vi "DrawSubMenuItems.vi"(7 "Collection in":refnum<class "Collection.lvclass">, 8 "error in (no error)":errorcluster, 9 "Coords":T2, 10 "Tag":string, 11 "Menu in":refnum<class "Menu.lvclass">) -> (0 "error out":errorcluster, 1 "SubMenu":bool, 2 "SelectedArea":T1, 3 "Menu out":refnum<class "Menu.lvclass">, 4 "SelectedItemTag":string, 5 "Collection out":refnum<class "Collection.lvclass">, 6 "GlobalArea":T1)   [LabVIEW 2021, in "Menu.lvlib" / "Menu.lvclass"]
uses:
  Menu.lvclass
  Menu.lvclass/Menu.ctl
  Picture2D/src/Collection/Collection.lvclass
  Picture2D/src/Rectangle/Rectangle.lvclass
  Picture2D/src/Text/Text.lvclass
  Picture2D/src/Picture/Image.lvclass
  Picture2D/src/Point/Point.lvclass
  C:/GitHub/Picture2D/src/Polygone/Polygone.lvclass
  C:/GitHub/Picture2D/src/Shape/Shape.lvclass
  C:/GitHub/Picture2D/src/Picture2D/Picture2D.lvclass
  C:/GitHub/Picture2D/src/IDrawable/IDrawable.lvclass
  C:/GitHub/Picture2D/src/IMovable/IMovable.lvclass
  C:/GitHub/Picture2D/src/IRotatable/IRotatable.lvclass
  C:/GitHub/Picture2D/src/IScalable/IScalable.lvclass
  C:/GitHub/Picture2D/src/Rectangle/Rectangle.lvclass
  C:/GitHub/Picture2D/src/Collection/Collection.lvclass
  C:/GitHub/Picture2D/src/Picture/Image.lvclass
  <vilib>/Utility/miscctls.llb/LVPoint32TypeDef.ctl
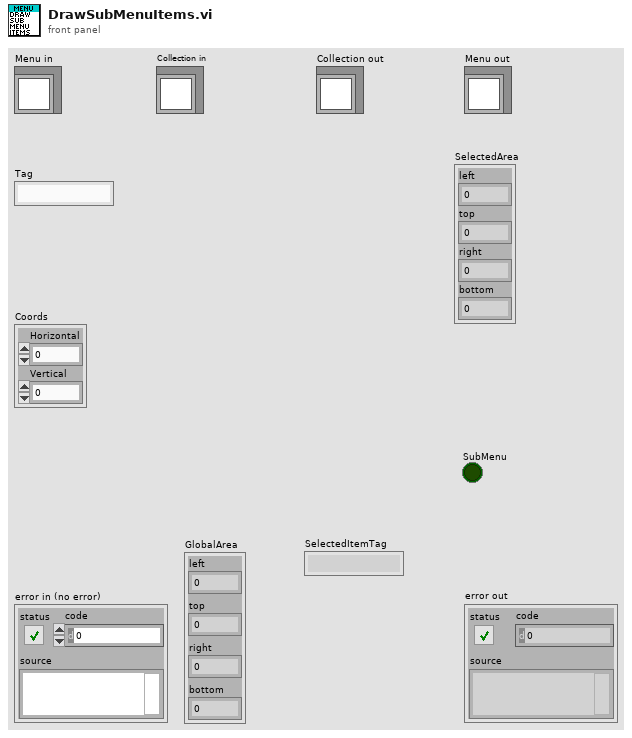
[diagram p1: front panel]
types:
  T1 = cluster{"left":i16, "top":i16, "right":i16, "bottom":i16}
  T2 = typedef "LVPoint32TypeDef.ctl" = cluster{"Horizontal":i32, "Vertical":i32}
  T3 = typedef "Menu.lvlib/Menu.lvclass/MenuItems.ctl" = cluster{"Item Name":string, "Short Cut":T4, "Checked":bool, "Enable":bool, "After item":string, "Item Tags":string[], "Item Names":string[], "Picture":refnum<class "Image.lvclass">, "Hilite Picture":refnum<class "Image.lvclass">, "Displayed":bool}
  T4 = typedef "LVMenuShortCut.ctl" = cluster{"Include Shift Key?":bool, "Include Ctrl Key?":bool, "Shortcut Key":string}
  T5 = typedef "Menu.lvlib/Menu.lvclass/MenuColors.ctl" = cluster{"Text":refnum<class "Color.lvclass">, "HiliteText":refnum<class "Color.lvclass">, "Background":refnum<class "Color.lvclass">, "BorderColor":refnum<class "Color.lvclass">, "Hilite":refnum<class "Color.lvclass">}
  T6 = enum16{"User-specified Font", "Application Font", "System Font", "Dialog Font"}
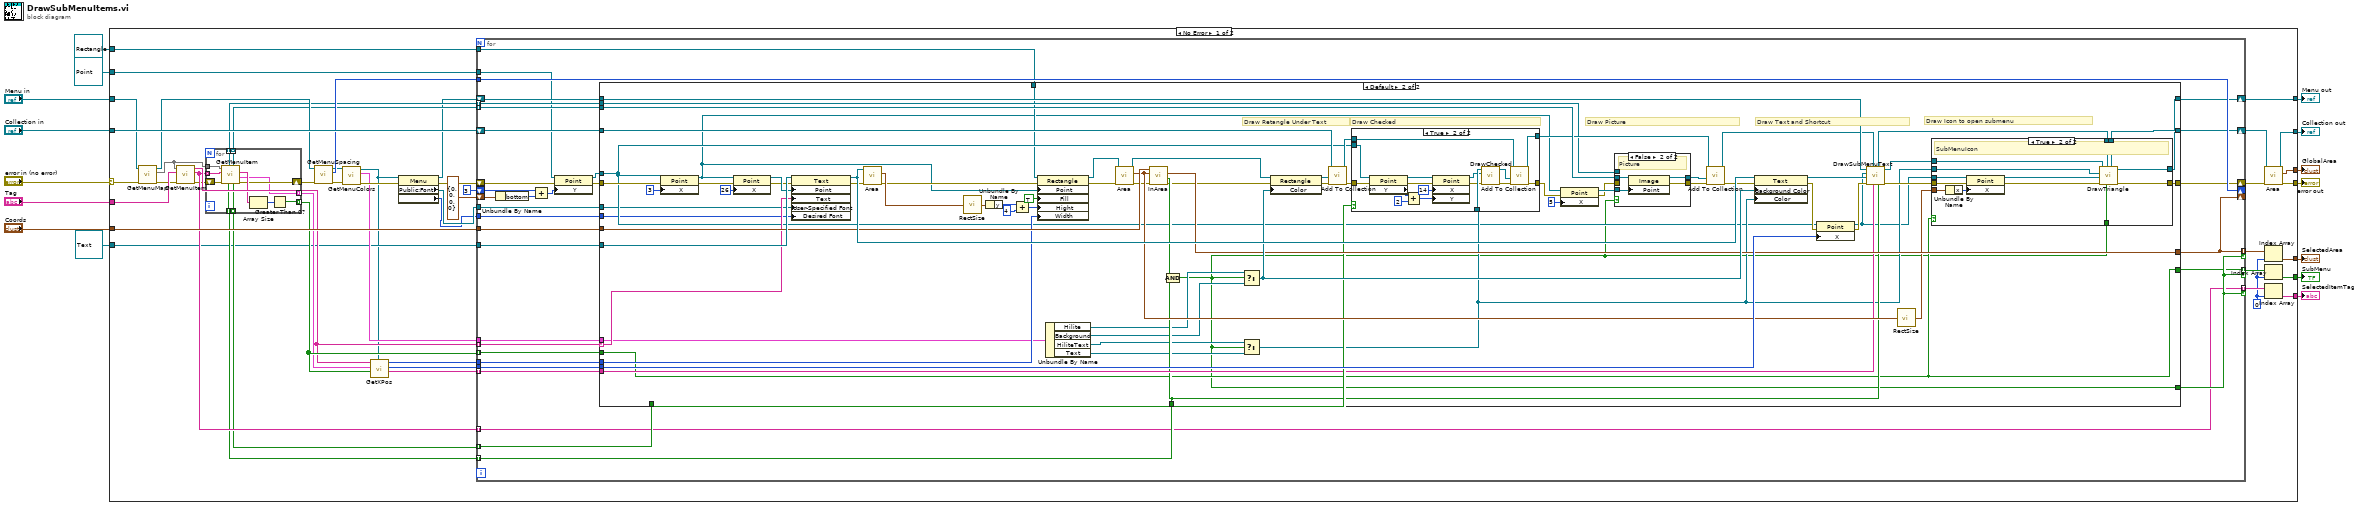
[diagram p0: block diagram]
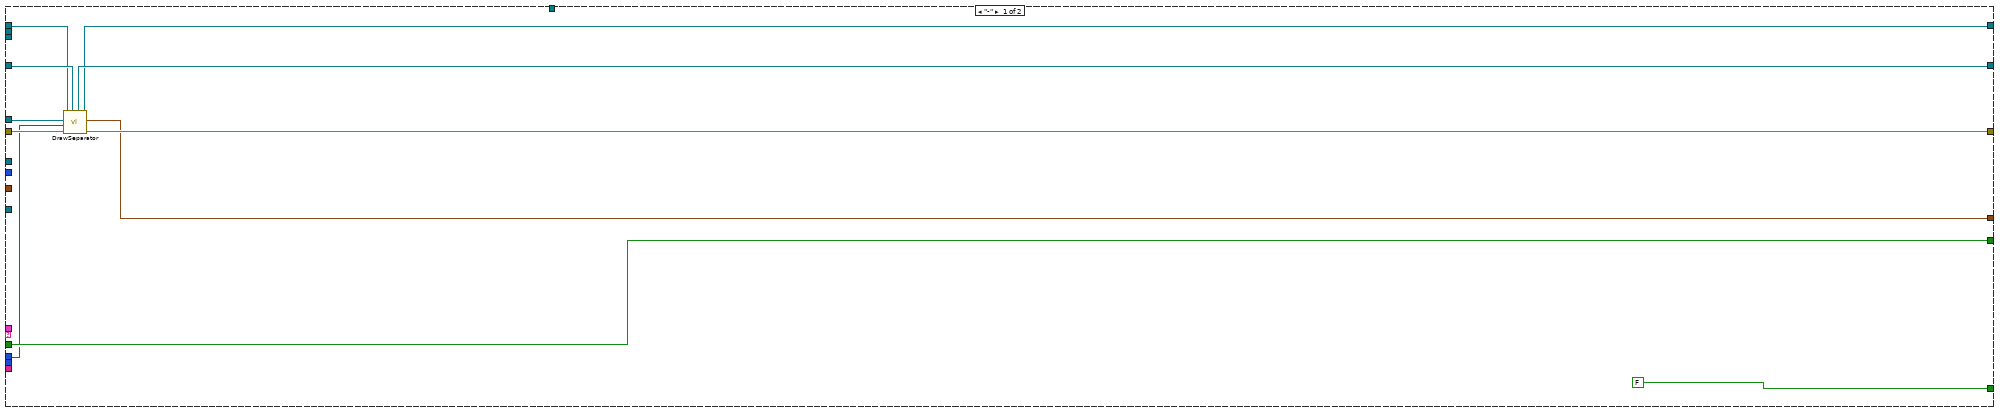
[diagram p2: hidden frame]
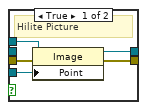
[diagram p3: hidden frame]
diagram:
  n1 = case shown="No Error" "error in (no error)" {
    selector: "error in (no error)" -> [w45 w237]
    tunnel: [w64 _] -> w15
    tunnel: [w62 _] -> w14
    tunnel: "Coords" -> [w58 _]
    tunnel: [w30 _] -> w12
    tunnel: [w51 _] -> w11
    tunnel: "Collection in" -> [w49 w238]
    tunnel: [w25 w238] -> w9
    tunnel: "Menu in" -> [w47 w239]
    tunnel: "Tag" -> [w43 _]
    tunnel: [w36 w237] -> w5
    tunnel: [w26 w239] -> w4
    tunnel: refnum<class "Text.lvclass"> refnum ("Picture2D.lvlib:Text") -> [w23 _]
    tunnel: refnum<class "Point.lvclass"> refnum ("reference") -> [w22 _]
    tunnel: refnum<class "Rectangle.lvclass"> refnum ("Rectangle") -> [w21 _]
    frame No Error {
      w52 = 0 ("index")
      n2 = call "GetMenuMap.vi"("error in (no error)"=w45, "Menu in"=w47) -> ("error out"=w40:errorcluster, "MenuMap"=w44:map{string, T3}, "Menu out"=w46:refnum<class "Menu.lvclass">)  [unwired: 7 in]
      n3 = call "GetMenuItem.vi"("error in (no error)"=w40, "Tag"=w43, "MenuMap"=w44) -> ("error out"=w39:errorcluster, "Item Tags"=w41:string[], "Item Names"=w42:string[])  [unwired: 1 in, 5 out]
      n4 = for {
        tunnel: w44 -> [w236]
        tunnel: w41 -> [w235] mode=indexing
        tunnel: [w232] -> w50 mode=indexing
        shift-right: [w230] -> w38
        shift-left: w39 -> [w231]
        tunnel: [w229] -> w35 mode=indexing
        tunnel: [w228] -> w34 mode=indexing
        tunnel: [w227] -> w33 mode=indexing
        tunnel: [w226] -> w32 mode=indexing
        tunnel: [w225] -> w31 mode=indexing
        n5 = call "GetMenuItem.vi"("error in (no error)"=w231, "Tag"=w235, "MenuMap"=w236) -> ("error out"=w230:errorcluster, "Short Cut"=w229:T4, "Item Tags"=w234:string[], "Checked"=w228:bool, "Picture"=w226:refnum<class "Image.lvclass">, "Enable"=w227:bool, "Hilite Picture"=w225:refnum<class "Image.lvclass">)  [unwired: 1 in, 1 out]
        n6 = Array Size(array=w234) -> (size(s)=w233:i32)
        n7 = Greater Than 0?(x=w233) -> (x > 0?=w232:bool)
      }
      n8 = call "GetMenuSpacing.vi"("error in (no error)"=w38, "Menu in"=w46) -> ("error out"=w37:errorcluster, "MenuSpacing"=w48:i32, "Menu out"=w29:refnum<class "Menu.lvclass">)  [unwired: 7 in]
      n9 = call "GetMenuColors.vi"("error in (no error)"=w37, "Menu in"=w29) -> ("error out"=w27:errorcluster, "MenuColors"=w24:T5, "Menu out"=w16:refnum<class "Menu.lvclass">)  [unwired: 7 in]
      n10 = call "GetXPos.vi"("Menu"=w16, "SubMenu"=w50, "Array"=w35, "Item Names"=w42) -> ("ShortCut Text"=w55:string[], "Start ShortCut"=w56:i16, "Total X"=w57:i16)  [unwired: 5 in]
      n11 = property class="Menu"(reference=w16, error in=w27) -> (reference out=w19:refnum<class "Menu.lvclass">, error out=w20:errorcluster, "Public:Font"=w18:refnum<class "Font.lvclass">, "Public:Desired Font"=w17:T6)
      n12 = for {
        tunnel: w42 -> [w90] mode=indexing
        shift-right: [w87] -> w54
        shift-left: w49 -> [w88]
        shift-right: [w89] -> _
        shift-left: T1 {"left"=0, "top"=0, "right"=0, "bottom"=0} ("Area out") -> [w96]
        tunnel: w58 -> [w92]
        shift-right: [w91] -> _
        shift-left: i16 3 ("Spacing") -> [w93]
        tunnel: w48 -> [w91]
        tunnel: [w72] -> w61 mode=indexing if=w82
        tunnel: [w89] -> w63 mode=indexing if=w82
        tunnel: w41 -> [w72] mode=indexing
        tunnel: w57 -> [w86]
        tunnel: w56 -> [w85]
        tunnel: w55 -> [w84] mode=indexing
        tunnel: w50 -> [w83] mode=indexing
        tunnel: [w73] -> w53 mode=indexing if=w82
        tunnel: w34 -> [w79] mode=indexing
        tunnel: w33 -> [w74] mode=indexing
        tunnel: w32 -> [w80] mode=indexing
        tunnel: w31 -> [w78] mode=indexing
        shift-right: [w77] -> w28
        shift-left: w20 -> [w76]
        shift-right: [w65] -> w26
        shift-left: w19 -> [w75]
        tunnel: w24 -> [w71]
        tunnel: w23 -> [w70]
        tunnel: w22 -> [w69]
        tunnel: w21 -> [w68]
        tunnel: w18 -> [w67]
        tunnel: w17 -> [w66]
        n13 = Unbundle By Name(w96) -> ("bottom"=w95:i16)
        n14 = Add(x=w93, y=w95) -> (x+y=w94:i32)
        n15 = property class="Point"(reference=w69, error in=w76, "Y"=w94) -> (reference out=w97:refnum<class "Point.lvclass">, error out=w81:errorcluster)
        n16 = case shown="Default" w90 {
          selector: w90 -> [_ w171]
          tunnel: w97 -> [w99 w131]
          tunnel: w92 -> [_ w174]
          tunnel: w70 -> [_ w180]
          tunnel: [w103 w164] -> w89
          tunnel: [FALSE ("InArea") w112] -> w82
          tunnel: w88 -> [w102 w156]
          tunnel: [w104 w110] -> w87
          tunnel: w86 -> [w101 w172]
          tunnel: w85 -> [_ w169]
          tunnel: w84 -> [_ w144]
          tunnel: w83 -> [w107 w141]
          tunnel: [w107 w141] -> w73
          tunnel: w81 -> [w106 w162]
          tunnel: w80 -> [_ w154]
          tunnel: w79 -> [_ w157]
          tunnel: w78 -> [_ w150]
          tunnel: [w105 w138] -> w77
          tunnel: w75 -> [w100 w146]
          tunnel: w74 -> [_ w142]
          tunnel: w71 -> [_ w129]
          tunnel: w68 -> [_ w124]
          tunnel: w67 -> [_ w116]
          tunnel: w66 -> [_ w115]
          tunnel: [w98 w109] -> w65
          frame "-" {
            n17 = call "DrawSeparator.vi"("Collection in"=w102, "error in (no error)"=w106, "XPos"=w101, "Point"=w99, "Menu in"=w100) -> ("error out"=w105:errorcluster, "rect"=w103:T1, "Menu out"=w98:refnum<class "Menu.lvclass">, "Collection out"=w104:refnum<class "Collection.lvclass">)  [unwired: 3 in]
          }
          frame Default {
            # "Draw Retangle Under Text"
            # "Draw Checked"
            # "Draw Picture"
            # "Draw Icon to open submenu"
            # "Draw Text and Shortcut"
            n18 = property class="Point"(reference=w131, error in=w162, "X"=i16 3 ("Point:x")) -> (reference out=w119:refnum<class "Point.lvclass">, error out=w123:errorcluster)
            n19 = property class="Point"(reference=w119, error in=w123, "X"=i16 26 ("Point:x")) -> (reference out=w179:refnum<class "Point.lvclass">, error out=w122:errorcluster)
            n20 = property class="Text"(reference=w180, error in=w122, "Point"=w179, "Text"=w171, "User-Specified Font"=w116, "Desired Font"=w115) -> (reference out=w181:refnum<class "Text.lvclass">, error out=w161:errorcluster)
            n21 = call-dynamic "Area.vi"("error in (no error)"=w161, "Text in"=w181) -> ("error out"=w160:errorcluster, "rect"=w173:T1)  [unwired: 7 in, 1 out]
            n22 = call <vilib>:"RectSize.vi"("rect"=w173) -> ("point"=w176:cluster{"x":i16, "y":i16})
            n23 = Unbundle By Name(w176) -> ("y"=w175:i16)
            n24 = Add(x=w175, y=i16 4) -> (x+y=w168:i16)
            n25 = property class="Rectangle"(reference=w124, error in=w160, "Point"=w119, "Fill"=TRUE, "Hight"=w168, "Width"=w172) -> (reference out=w121:refnum<class "Rectangle.lvclass">, error out=w159:errorcluster)
            n26 = Unbundle By Name(w129) -> ("Hilite"=w125:refnum<class "Color.lvclass">, "Background"=w126:refnum<class "Color.lvclass">, "HiliteText"=w128:refnum<class "Color.lvclass">, "Text"=w127:refnum<class "Color.lvclass">)
            n27 = call-dynamic "Area.vi"("error in (no error)"=w159, "Rectangle in"=w121) -> ("error out"=w158:errorcluster, "rect"=w163:T1, "Rectangle out"=w120:refnum<class "Rectangle.lvclass">)  [unwired: 7 in]
            n28 = call "InArea.vi"("error in (no error)"=w158, "Area in"=w163, "Coords"=w174) -> ("error out"=w133:errorcluster, "InArea"=w151:bool, "Area out"=w164:T1)  [unwired: 6 in]
            n29 = Compound Arithmetic op=AND(w151, w142) -> (w112:bool)
            n30 = Select(t=w125, s=w112, f=w126) -> (s? t:f=w166:refnum<class "Color.lvclass">)
            n31 = Select(t=w128, s=w112, f=w127) -> (s? t:f=w132:refnum<class "Color.lvclass">)
            n32 = property class="Rectangle"(reference=w120, error in=w133, "Color"=w166) -> (reference out=w170:refnum<class "Rectangle.lvclass">, error out=w147:errorcluster)
            n33 = call-dynamic "Add To Collection.vi"("error in (no error)"=w147, "IDrawable"=w170, "Collection in"=w156) -> ("error out"=w130:errorcluster, "Collection out"=w155:refnum<class "Collection.lvclass">)  [unwired: 7 in]
            n34 = case shown="True" w157 {
              tunnel: [w192 w208] -> w152
              tunnel: w155 -> [w192 w207]
              tunnel: [w191 w206] -> w118
              tunnel: w130 -> [w191 w195]
              tunnel: w132 -> [_ w205]
              tunnel: w131 -> [_ w193]
              frame False {
              }
              frame True {
                n35 = property class="Point"(reference=w193, error in=w195) -> (reference out=w201:refnum<class "Point.lvclass">, error out=w194:errorcluster, "Y"=w202:i16)
                n36 = Add(x=w202, y=i16 2) -> (x+y=w203:i16)
                n37 = property class="Point"(reference=w201, error in=w194, "X"=i16 14 ("Point:x"), "Y"=w203) -> (reference out=w198:refnum<class "Point.lvclass">, error out=w197:errorcluster)
                n38 = call "DrawChecked.vi"("error in"=w197, "Point"=w198, "Color"=w205) -> ("error out"=w196:errorcluster, "Collection out"=w204:refnum<class "Collection.lvclass">)  [unwired: 7 in]
                n39 = call-dynamic "Add To Collection.vi"("error in (no error)"=w196, "IDrawable"=w204, "Collection in"=w207) -> ("error out"=w206:errorcluster, "Collection out"=w208:refnum<class "Collection.lvclass">)  [unwired: 7 in]
              }
            }
            n40 = property class="Point"(reference=w119, error in=w118, "X"=i16 5 ("Point:x")) -> (reference out=w149:refnum<class "Point.lvclass">, error out=w117:errorcluster)
            n41 = case shown="False" w112 {
              tunnel: w154 -> [_ w188]
              tunnel: [w186 w190] -> w153
              tunnel: w149 -> [w185 w189]
              tunnel: w150 -> [w184 _]
              tunnel: [w183 w187] -> w134
              tunnel: w117 -> [w182 _]
              frame True {
                # "Hilite Picture"
                n42 = property class="Image"(reference=w184, error in=w182, "Point"=w185) -> (reference out=w186:refnum<class "Image.lvclass">, error out=w183:errorcluster)
              }
              frame False {
                # "Picture"
                n43 = property class="Image"(reference=w188, "Point"=w189) -> (reference out=w190:refnum<class "Image.lvclass">, error out=w187:errorcluster)  [unwired: 1 in]
              }
            }
            n44 = call-dynamic "Add To Collection.vi"("error in (no error)"=w134, "IDrawable"=w153, "Collection in"=w152) -> ("error out"=w137:errorcluster, "Collection out"=w143:refnum<class "Collection.lvclass">)  [unwired: 7 in]
            n45 = property class="Text"(reference=w181, error in=w137, "Background Color"=w166, "Color"=w132) -> (reference out=w145:refnum<class "Text.lvclass">, error out=w136:errorcluster)
            n46 = property class="Point"(reference=w131, error in=w136, "X"=w169) -> (reference out=w113:refnum<class "Point.lvclass">, error out=w135:errorcluster)
            n47 = call "DrawSubMenuText.vi"("Enable"=w142, "ShortcutText"=w144, "Collection in"=w143, "error in (no error)"=w135, "Text"=w145, "InsertionPoint"=w113, "Menu in"=w146) -> ("error out"=w139:errorcluster, "Menu out"=w114:refnum<class "Menu.lvclass">, "Collection out"=w111:refnum<class "Collection.lvclass">)  [unwired: 2 in]
            n48 = call <vilib>:"RectSize.vi"("rect"=w163) -> ("point"=w140:cluster{"x":i16, "y":i16})
            n49 = case shown="True" w141 {
              tunnel: w132 -> [_ w214]
              tunnel: [w211 w220] -> w138
              tunnel: w140 -> [_ w223]
              tunnel: w113 -> [_ w222]
              tunnel: w139 -> [w211 w221]
              tunnel: w114 -> [w209 w215]
              tunnel: w112 -> [_ w216]
              tunnel: w111 -> [w210 w218]
              tunnel: [w210 w217] -> w110
              tunnel: [w209 w212] -> w109
              frame False {
                # "No Triangle"
              }
              frame True {
                # "SubMenuIcon"
                n50 = Unbundle By Name(w223) -> ("x"=w224:i16)
                n51 = property class="Point"(reference=w222, error in=w221, "X"=w224) -> (reference out=w213:refnum<class "Point.lvclass">, error out=w219:errorcluster)
                n52 = call "DrawTriangle.vi"("Open?"=w216, "Collection in"=w218, "error in"=w219, "Point"=w213, "Color"=w214, "Menu in"=w215) -> ("error out"=w220:errorcluster, "Menu out"=w212:refnum<class "Menu.lvclass">, "Collection out"=w217:refnum<class "Collection.lvclass">)  [unwired: 3 in]
              }
            }
          }
        }
      }
      n53 = call-dynamic "Area.vi"("error in (no error)"=w28, "Collection in"=w54) -> ("error out"=w36:errorcluster, "Area"=w30:T1, "Collection out"=w25:refnum<class "Collection.lvclass">)  [unwired: 7 in]
      n54 = Index Array(array=w63, index=w52) -> (element=w64:T1)
      n55 = Index Array(array=w53, index=w52) -> (element=w51:bool)
      n56 = Index Array(array=w61, index=w52) -> (element=w62:string)
    }
    frame Error {
    }
  }
  "error out" <- w5
  "Menu out" <- w4
  "SelectedArea" <- w15
  "SelectedItemTag" <- w14
  "GlobalArea" <- w12
  "SubMenu" <- w11
  "Collection out" <- w9
